vi "Write Base Path.vi"(8 "error in (no error)":errorcluster, 10 "Base Path":path, 11 "StorageService in":refnum<class "StorageService.lvclass">) -> (0 "error out":errorcluster, 3 "StorageService out":refnum<class "StorageService.lvclass">)   [LabVIEW 2014, in "StorageService.lvclass"]
uses:
  StorageService.lvclass
  StorageService.lvclass/StorageService.ctl
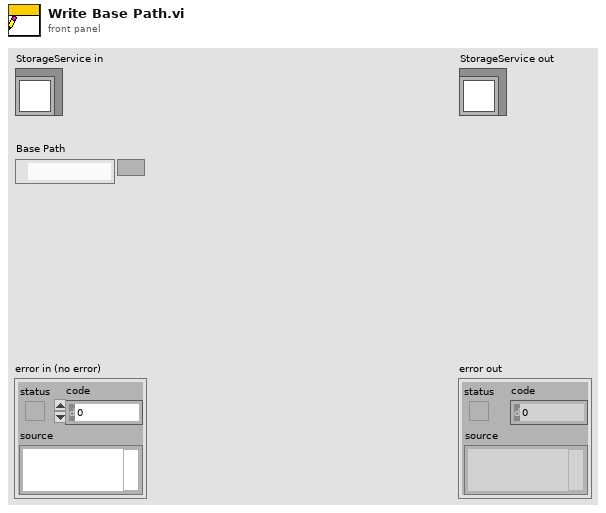
[diagram p1: front panel]
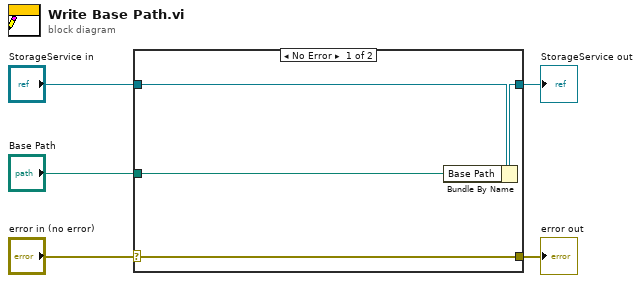
[diagram p0: block diagram]
diagram:
  n1 = case shown="No Error" "error in (no error)" {
    selector: "error in (no error)" -> [w9 w10]
    tunnel: [w9 w10] -> w4
    tunnel: [w7 w11] -> w2
    tunnel: "StorageService in" -> [w8 w11]
    tunnel: "Base Path" -> [w6 _]
    frame No Error {
      n2 = Bundle By Name(cluster=w8, "Base Path"=w6) -> (w7:refnum<class "StorageService.lvclass">)
    }
    frame Error {
    }
  }
  "error out" <- w4
  "StorageService out" <- w2
